vi "CB Solve DARE.vi"(6 "epsilon":dbl, 8 "R":T1, 9 "Q":T1, 10 "B":T1, 11 "A":T1) -> (3 "X":T1)   [LabVIEW 2020]
uses:
  <vilib>/Analysis/Matrix/Datatypes/RealMatrix.ctl
  <vilib>/Analysis/7linalg.llb/Real Transpose Matrix.vi
  <vilib>/Analysis/baseanly.llb/Real A x B.vi
  <vilib>/Analysis/_algsub.llb/Real Matrix Norm.vi
  <vilib>/Analysis/baseanly.llb/Real Inverse Matrix.vi
  <vilib>/Analysis/7linalg.llb/Create Special Real Matrix.vi
  <vilib>/Analysis/Matrix/Numeric/Add/Add - RM,RM.vi
  <vilib>/Analysis/NI_AALBase.lvlib
  <vilib>/Analysis/NI_AALPro.lvlib
  <vilib>/Analysis/Matrix/NI_Matrix.lvlib
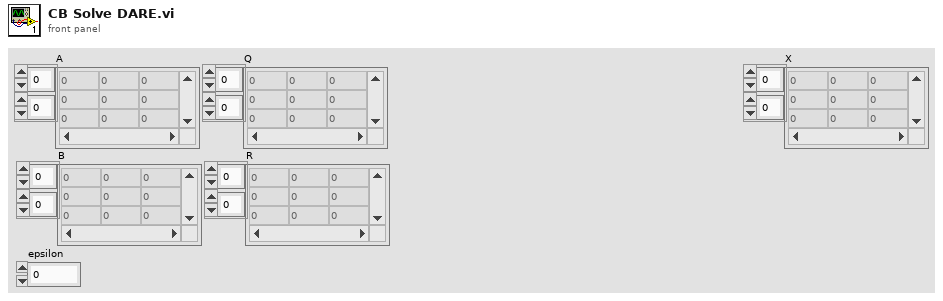
[diagram p1: front panel]
types:
  T1 = typedef "NI_Matrix.lvlib/RealMatrix.ctl" = dbl[][]
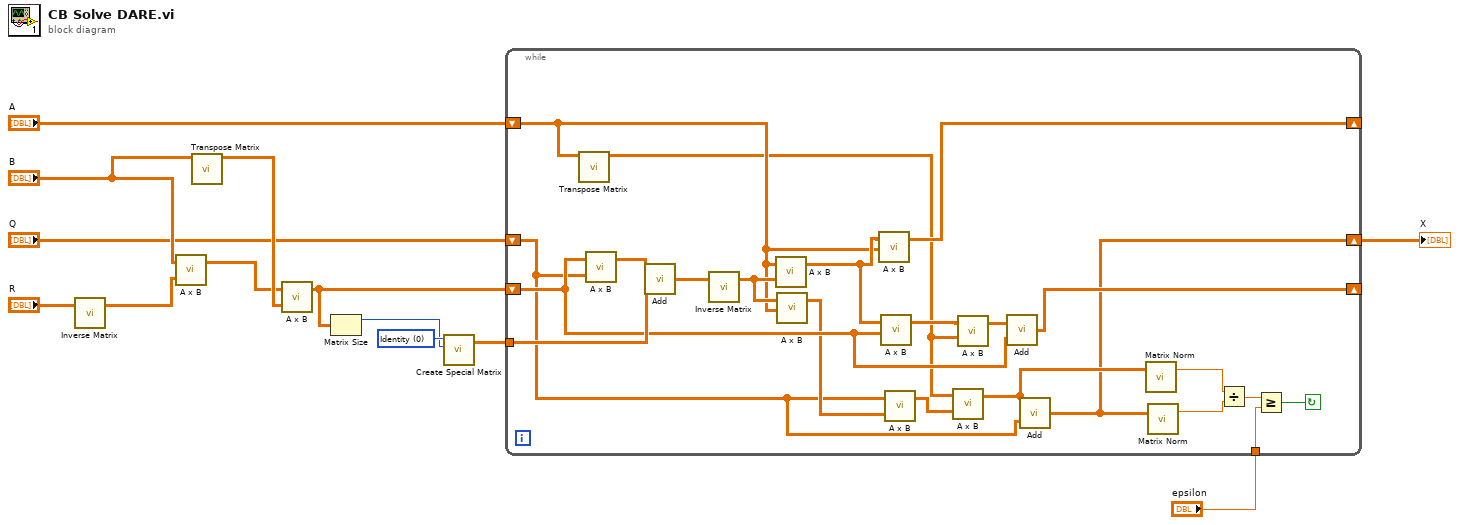
[diagram p0: block diagram]
diagram:
  w7 = 0 items=["Identity", "Diagonal", "Toeplitz", "Vandermonde", "Companion", "Hankel", "Hadamard", "Wilkinson", "Hilbert", "Inverse Hilbert", "Rosser", "Pascal"] ("matrix type")
  n1 = call-poly <vilib>:"Inverse Matrix.vi"("Input Matrix"="R") -> ("Inverse Matrix"=w3:T1)  [unwired: 1 in, 1 out]
  n2 = call-poly <vilib>:"A x B.vi"("B"=w3, "A"="B") -> ("A x B"=w11:T1)  [unwired: 1 out]
  n3 = call-poly <vilib>:"Transpose Matrix.vi"("Input Matrix"="B") -> ("Matrix Transpose"=w12:T1)  [unwired: 9 in, 1 out]
  n4 = call-poly <vilib>:"A x B.vi"("B"=w12, "A"=w11) -> ("A x B"=w8:T1)  [unwired: 1 out]
  n5 = Matrix Size(0:w8) -> (1:w6:i32)  [unwired: 1 out]
  n6 = call-poly <vilib>:"Create Special Matrix.vi"("matrix type"=w7, "matrix size"=w6) -> ("Special Matrix"=w5:T1)  [unwired: 3 in, 1 out]
  n7 = while {
    shift-right: [w32] -> _
    shift-left: "A" -> [w25]
    shift-right: [w27] -> _
    shift-left: w8 -> [w28]
    shift-right: [w14] -> w1
    shift-left: "Q" -> [w21]
    tunnel: w5 -> [w34]
    tunnel: "epsilon" -> [w16]
    stop <- w15 continue-if-true
    n8 = call-poly <vilib>:"Transpose Matrix.vi"("Input Matrix"=w25) -> ("Matrix Transpose"=w22:T1)  [unwired: 9 in, 1 out]
    n9 = call-poly <vilib>:"A x B.vi"("B"=w21, "A"=w28) -> ("A x B"=w35:T1)  [unwired: 1 out]
    n10 = call-poly <vilib>:"Add.vi"("Real Matrix B"=w34, "Real Matrix A"=w35) -> ("A + B"=w33:T1)
    n11 = call-poly <vilib>:"Inverse Matrix.vi"("Input Matrix"=w33) -> ("Inverse Matrix"=w26:T1)  [unwired: 1 in, 1 out]
    n12 = call-poly <vilib>:"A x B.vi"("B"=w26, "A"=w25) -> ("A x B"=w31:T1)  [unwired: 1 out]
    n13 = call-poly <vilib>:"A x B.vi"("B"=w25, "A"=w26) -> ("A x B"=w24:T1)  [unwired: 1 out]
    n14 = call-poly <vilib>:"A x B.vi"("B"=w25, "A"=w31) -> ("A x B"=w32:T1)  [unwired: 1 out]
    n15 = call-poly <vilib>:"A x B.vi"("B"=w28, "A"=w31) -> ("A x B"=w30:T1)  [unwired: 1 out]
    n16 = call-poly <vilib>:"A x B.vi"("B"=w24, "A"=w21) -> ("A x B"=w23:T1)  [unwired: 1 out]
    n17 = call-poly <vilib>:"A x B.vi"("B"=w23, "A"=w22) -> ("A x B"=w20:T1)  [unwired: 1 out]
    n18 = call-poly <vilib>:"A x B.vi"("B"=w22, "A"=w30) -> ("A x B"=w29:T1)  [unwired: 1 out]
    n19 = call-poly <vilib>:"Add.vi"("Real Matrix B"=w28, "Real Matrix A"=w29) -> ("A + B"=w27:T1)
    n20 = call-poly <vilib>:"Add.vi"("Real Matrix B"=w21, "Real Matrix A"=w20) -> ("A + B"=w14:T1)
    n21 = call-poly <vilib>:"Matrix Norm.vi"("Input Matrix"=w20) -> ("norm"=w19:dbl)  [unwired: 1 in, 1 out]
    n22 = call-poly <vilib>:"Matrix Norm.vi"("Input Matrix"=w14) -> ("norm"=w18:dbl)  [unwired: 1 in, 1 out]
    n23 = Divide(x=w19, y=w18) -> (x/y=w17:dbl)
    n24 = Greater Or Equal?(x=w17, y=w16) -> (x >= y?=w15:bool)
  }
  "X" <- w1
